vi "Copy to Clipboard.vi"(4 "error in (no error)":errorcluster, 6 "Format (CF_TEXT)":T1, 7 "string in":string) -> (0 "error out":errorcluster)   [LabVIEW 2011]
doc: "This VI either reads a text string from the clipboard from the OS or writes a text string to this clipboard.\n\nIf there is no text available in the clipboard the VI returns an empty string.\nWhen calling this VI with the operation to put a text to the clipboard and the string is not empty, this VI will clear anything else in the clipboard before writing the string into the clipboard.\n\n© 1997 Electronic Application Systems, Netherlands\nAll rights reserved.\n\nAddress:\nElectronic Application Systems, Rolf Kalbermatter\nBongerd 235, 2906 VG Capelle a/d IJssel, Netherlands\nTel: +31 (0)10 442 0905\nemail: rkalbermatter@compuserve.com"
uses:
  Clipboard Formats.ctl
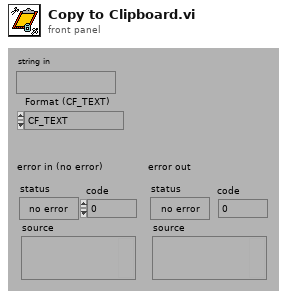
[diagram p1: front panel]
types:
  T1 = typedef "Clipboard Formats.ctl" = enum16{"CF_TEXT"}
  T2 = enum16{"GMEM_FIXED", "GMEM_MOVEABLE", "GMEM_NOCOMPACT", "GMEM_NODISCARD", "GMEM_ZEROINIT", "GMEM_MODIFY", "GMEM_DISCARDABLE", "GMEM_NOT_BANKED", "GMEM_SHARE", "GMEM_DDESHARE", "GMEM_NOTIFY", "GMEM_LOWER", "GMEM_VALID_FLAGS", "GMEM_INVALID_HANDLE", "GHND", "GPTR"}
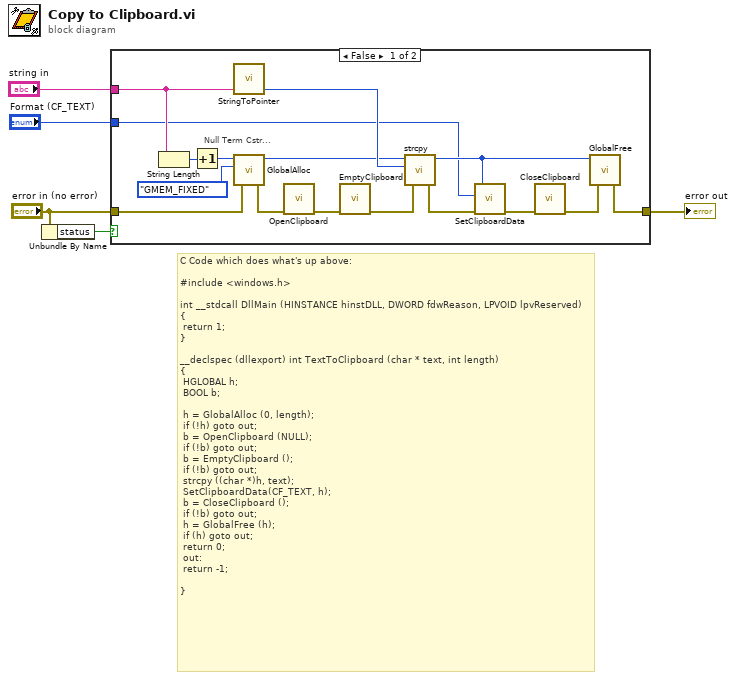
[diagram p0: block diagram]
diagram:
  # "C Code which does what's up above:\n\n#include <windows.h>\n\nint __stdcall DllMain (HINSTANCE hinstDLL, DWORD fdwReason, LPVOID lpvReserved)\n{\n\treturn 1;\n}\n\n__declspec (dllexport) int TextToClipboard (char * text, int length)\n{\n\tHGLOBAL h;\n\tBOOL b;\n\n\th = GlobalAlloc (0, length);\n\tif (!h) goto out;\n\tb = OpenClipboard (NULL);\n\tif (!b) goto out;\n\tb = EmptyClipboard ();\n\tif (!b) goto out;\n\tstrcpy ((char *)h, text);\n\tSetClipboardData(CF_TEXT, h);\n\tb = CloseClipboard ();\n\tif (!b) goto out;\n\th = GlobalFree (h);\n\tif (h) goto out;\n\treturn 0;\n\tout:\n\treturn -1;\n\t\n}"
  n1 = Unbundle By Name("error in (no error)") -> ("status"=w5:bool)
  n2 = case shown="False" w5 {
    tunnel: "error in (no error)" -> [w18 w22]
    tunnel: "string in" -> [w11 _]
    tunnel: [w15 w22] -> w2
    tunnel: "Format (CF_TEXT)" -> [w6 _]
    frame False {
      # "Null Term Cstr..."
      n3 = String Length(string=w11) -> (length=w17:i32)
      n4 = Increment(x=w17) -> (x+1=w10:i32)
      n5 = call "StringToPointer.vi"("string"=w11) -> ("pointer"=w12:i32)  [unwired: 4 out]
      n6 = call "GlobalAlloc.vi"("error in (no error)"=w18, "uFlags"=T2."GMEM_FIXED", "Bytes (0)"=w10) -> ("error out"=w19:errorcluster, "hMem"=w9:i32)  [unwired: 3 out]
      n7 = call "OpenClipboard.vi"("error in (no error)"=w19) -> ("error out"=w21:errorcluster)  [unwired: 6 out]
      n8 = call "EmptyClipboard.vi"("error in (no error)"=w21) -> ("error out"=w14:errorcluster)  [unwired: 6 out]
      n9 = call "strcpy.vi"("error in (no error)"=w14, "lpString2 (NULL)\n[SOURCE]"=w12, "lpString1 (NULL)\n[TARGET]"=w9) -> ("error out"=w13:errorcluster, "lpString1"=w8:i32)  [unwired: 3 out]
      n10 = call "SetClipboardData.vi"("error in (no error)"=w13, "Format (CF_TEXT)"=w6, "hMem"=w8) -> ("error out"=w20:errorcluster)  [unwired: 4 out]
      n11 = call "CloseClipboard.vi"("error in (no error)"=w20) -> ("error out"=w16:errorcluster)  [unwired: 6 out]
      n12 = call "GlobalFree.vi"("error in (no error)"=w16, "hMem (NULL)"=w8) -> ("error out"=w15:errorcluster)  [unwired: 5 out]
    }
    frame True {
    }
  }
  "error out" <- w2
